vi "Get Security Level.vi"(1 "Security System.lvclass":refnum<class "Security System.lvclass">) -> (0 "Current Level":T1)   [LabVIEW 2020, in "Security System.lvclass"]
uses:
  Security System.lvclass
  Security Level.ctl
  Security System.lvclass/Security System.ctl
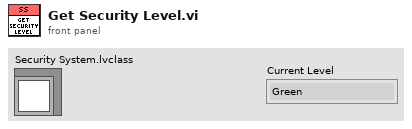
[diagram p1: front panel]
types:
  T1 = typedef "Security System.lvclass/Security Level.ctl" = enum16{"Green", "Yellow", "Orange", "Red"}
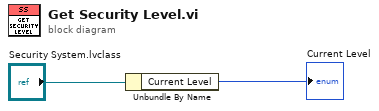
[diagram p0: block diagram]
diagram:
  n1 = Unbundle By Name("Security System.lvclass") -> ("Current Level"=→"Current Level":T1)
